vi "Configure Calibration ENR Table.vi"(0 "VISA resource name":refnum<visa-resource-name>, 5 "ID for Calibration ENR Table":string, 7 "Serial Number for Calibration ENR Table":string, 9 "Calibration ENR Table Data Entry (Frequency/Amplitude)":dbl[][](array[numeric]), 11 "error in (no error)":errorcluster) -> (4 "VISA resource name out":refnum<visa-resource-name>, 15 "error out":errorcluster)   [LabVIEW 2014, in "Agilent ESA PSA Series.lvlib"]
doc: "Configures the calibration table settings of the Noise Figure personality.\n\n<B>Note:</B> \n\nThis VI is only valid in Noise Figure personality. Use <B>Switch Personality</B> VI to switch to Noise Figure before calling this VI."
uses:
  Agilent ESA PSA Series.lvlib
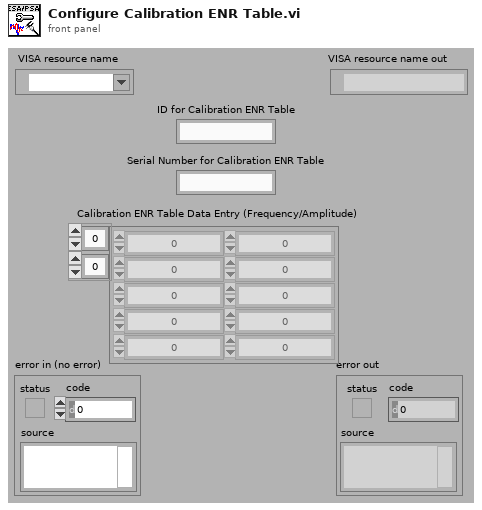
[diagram p1: front panel]
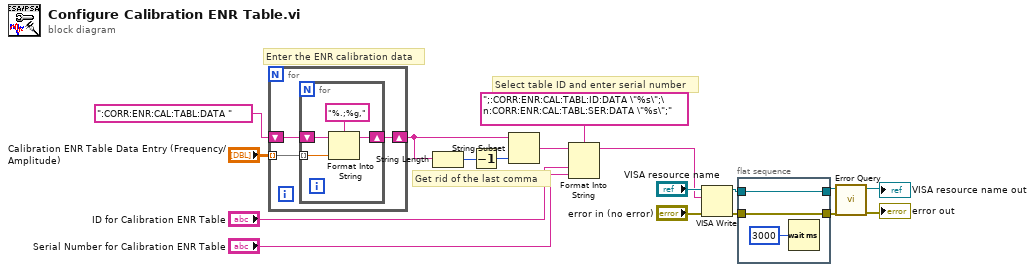
[diagram p0: block diagram]
diagram:
  # "Get rid of the last comma"
  # "Select table ID and enter serial number"
  # "Enter the ENR calibration data"
  n1 = for {
    tunnel: "Calibration ENR Table Data Entry (Frequency/Amplitude)" -> [w21] mode=indexing
    shift-right: [w19] -> w12
    shift-left: ":CORR:ENR:CAL:TABL:DATA " -> [w20]
    n2 = for {
      tunnel: w21 -> [w25] mode=indexing
      shift-right: [w23] -> w19
      shift-left: w20 -> [w24]
      n3 = Format Into String(format string="%.;%g,", initial string=w24, w25) -> (resulting string=w23:string)  [unwired: 1 in, 1 out]
    }
  }
  n4 = String Length(string=w12) -> (length=w13:i32)
  n5 = Decrement(x=w13) -> (x-1=w14:i32)
  n6 = String Subset(string=w12, length (rest)=w14) -> (substring=w7:string)  [unwired: 1 in]
  n7 = Format Into String(format string=";:CORR:ENR:CAL:TABL:ID:DATA \"%s\";\n:CORR:ENR:CAL:TABL:SER:DATA \"%s\";", initial string=w7, "ID for Calibration ENR Table", "Serial Number for Calibration ENR Table") -> (resulting string=w8:string)  [unwired: 1 in, 1 out]
  n8 = VISA Write(VISA resource name="VISA resource name", write buffer=w8, error in (no error)="error in (no error)") -> (VISA resource name out=w4:refnum<visa-resource-name>, error out=w2:errorcluster)  [unwired: 1 out]
  n9 = flat-sequence {
    tunnel: w4 -> [w27]
    tunnel: [w27] -> w3
    tunnel: w2 -> [w26]
    tunnel: [w26] -> w1
    frame #0 {
      n10 = Wait (ms)(milliseconds to wait=u32 3000) -> ()  [unwired: 1 out]
    }
  }
  n11 = call "Error Query.vi"("error in (no error)"=w1, "VISA resource name"=w3) -> ("error out"=→"error out":errorcluster, "VISA resource name out"=→"VISA resource name out":refnum<visa-resource-name>)  [unwired: 6 in, 2 out]
